vi "PMBus Block Process Call.vi"(0 "DevType":i32, 1 "CommandCode":u8, 2 "WriteByteCount":u8, 5 "DevIndex":i32, 7 "PMBusIndex":i32, 9 "SlaveAddr":u8, 12 "pWriteData":u8[](array[numeric]), 13 "PEC":u8) -> (4 "pReadData":u8[](array[numeric]), 6 "pReadByteCount":u8, 8 "function return":i32)   [LabVIEW 2010, in "ControlPMBus.lvlib"]
doc: "int WINAPI PMBus_BlockProcessCall(int DevType,int DevIndex,int PMBusIndex,unsigned char SlaveAddr,unsigned char CommandCode,unsigned char *pWriteData,unsigned char WriteByteCount,unsigned char *pReadData,unsigned char *pReadByteCount,unsigned char PEC);"
uses:
  ControlPMBus.lvlib
  ControlPMBus/Ginkgo_Driver.dll
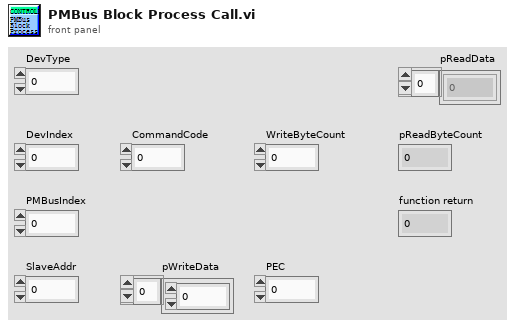
[diagram p1: front panel]
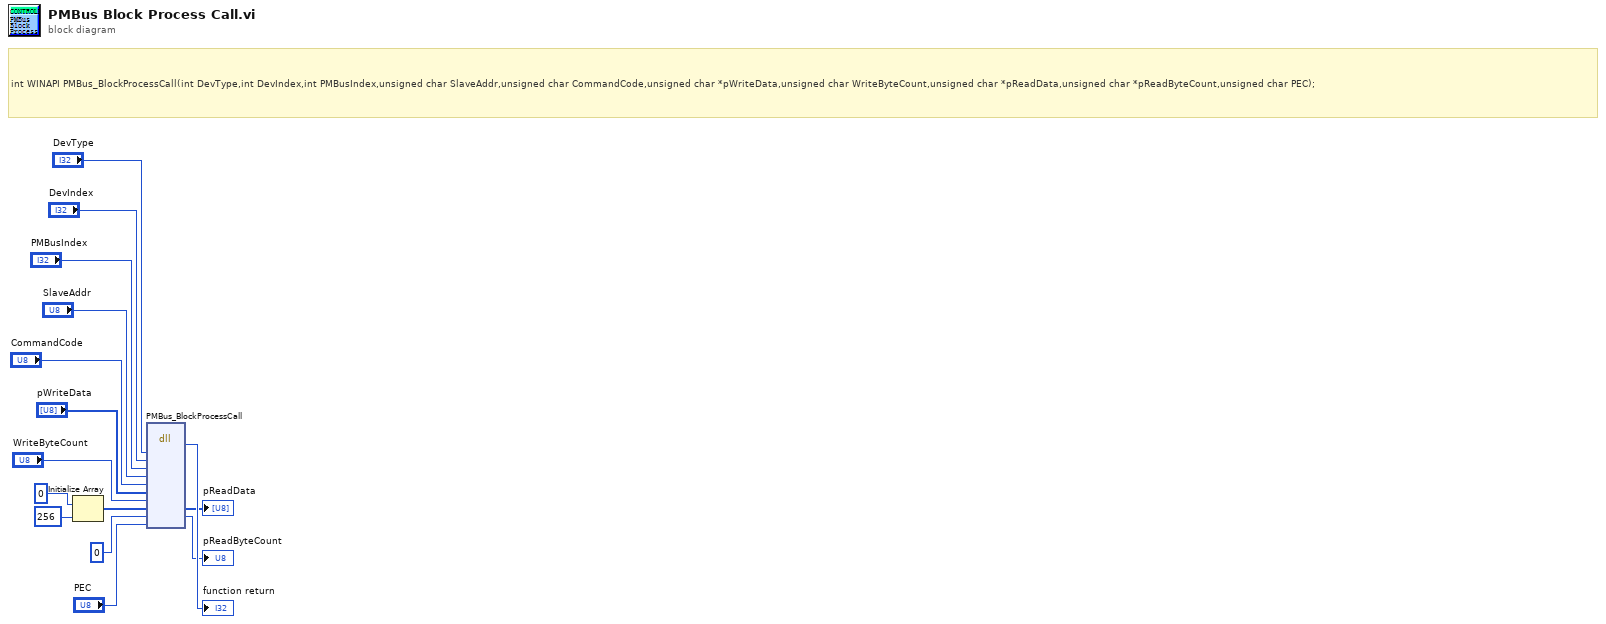
[diagram p0: block diagram]
diagram:
  # "int WINAPI PMBus_BlockProcessCall(int DevType,int DevIndex,int PMBusIndex,unsigned char SlaveAddr,unsigned char CommandCode,unsigned char *pWriteData,unsigned char WriteByteCount,unsigned char *pReadData,unsigned char *pReadByteCount,unsigned char PEC);"
  n1 = Initialize Array(u8 0 ("element"), 256 ("dimension size")) -> (w7:u8[])
  n2 = dll-call lib="E:/Project/vt_ginkgo/truck/Ginkgo Driver/vs2010/Ginkgo_USB-I2C&SPI&CAN_API_v2.0.3.3/lib/labview_32bit/ControlPMBus/Ginkgo_Driver.*" fn="PMBus_BlockProcessCall"("DevType"="DevType", "DevIndex"="DevIndex", "PMBusIndex"="PMBusIndex", "SlaveAddr"="SlaveAddr", "CommandCode"="CommandCode", "pWriteData"="pWriteData", "WriteByteCount"="WriteByteCount", "pReadData"=w7, "pReadByteCount"=u8 0, "PEC"="PEC") -> (→"function return":i32, "pReadData"=→"pReadData":u8[], "pReadByteCount"=→"pReadByteCount":u8)  [unwired: 11 in, 2 out]
